vi "uMsg_Delayed Create.vi"(6 "# of times (1)":i32=1, 8 "error in (no error)":errorcluster, 9 "delay (ms)":i32, 10 "Msg":refnum<class "uMsg.lvclass">, 11 "Destination":refnum<class "uTransport.lvclass">) -> (0 "error out":errorcluster, 3 "uMsg_Delayed out":refnum<class "uMsg_Delayed.lvclass">)   [LabVIEW 2023, in "uFramework.lvlib" / "uMsg_Delayed.lvclass"]
uses:
  uMsg_Delayed.lvclass
  uTransport/uTransport.lvclass
  uMsg/uMsg.lvclass
  uMsg_Delayed.lvclass/uMsg_Delayed.ctl
  uMsg_Delayed Daemon.vi
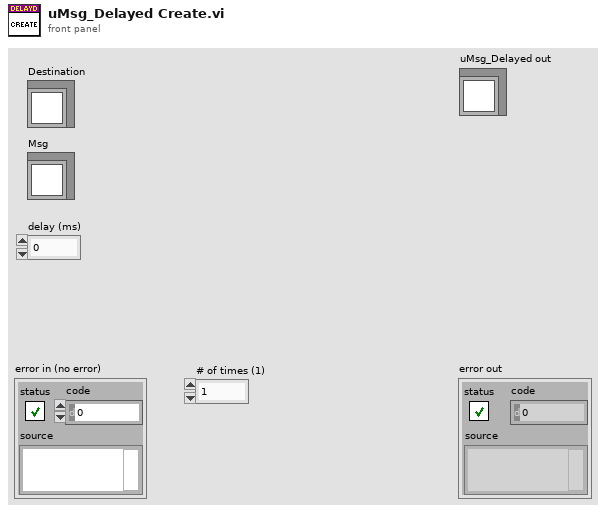
[diagram p1: front panel]
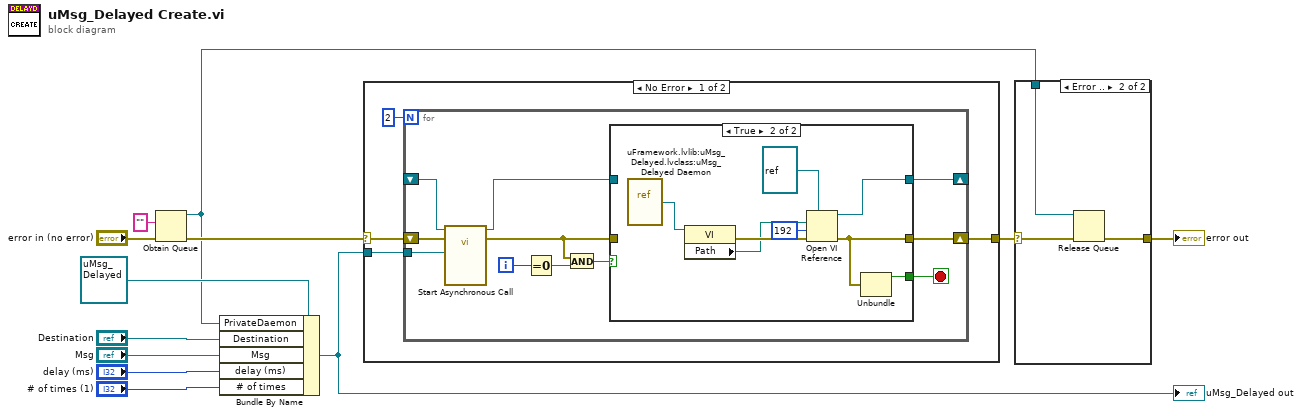
[diagram p0: block diagram]
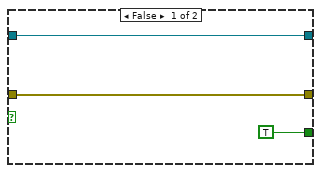
[diagram p3: hidden frame]
diagram:
  n1 = Obtain Queue(element data type="" ("Msg"), error in (no error)="error in (no error)") -> (queue out=w2:refnum<queue>, error out=w12:errorcluster)  [unwired: 3 in, 1 out]
  n2 = Bundle By Name(cluster=refnum<class "uMsg_Delayed.lvclass"> refnum ("uMsg_Delayed in"), "PrivateDaemon"=w2, "Destination"="Destination", "Msg"="Msg", "delay (ms)"="delay (ms)", "# of times"="# of times (1)") -> (w1:refnum<class "uMsg_Delayed.lvclass">)
  "uMsg_Delayed out" <- w1
  n3 = case shown="No Error" w12 {
    selector: w12 -> [w14 w39]
    tunnel: [w16 w39] -> w4
    tunnel: w1 -> [w13 _]
    frame No Error {
      n4 = for {
        N: 2 -> [_]
        shift-right: [w24] -> w16
        shift-left: w14 -> [w27]
        shift-right: [w25] -> _
        shift-left: _ -> [w26]
        tunnel: w13 -> [w17]
        i -> [w23]
        stop <- w18 stop-if-true
        n5 = call-by-ref "Start Asynchronous Call"(reference=w26, error in=w27, "uMsg_Delayed in"=w17) -> (reference out=w22:refnum<vi>, error out=w19:errorcluster)  [unwired: 11 in]
        n6 = Equal To 0?(x=w23) -> (x = 0?=w20:bool)
        n7 = And(x=w19, y=w20) -> (x .and. y?=w21:bool)
        n8 = case shown="True" w21 {
          tunnel: w19 -> [w29 _]
          tunnel: [w30 w34] -> w25
          tunnel: [w29 w33] -> w24
          tunnel: w22 -> [w30 _]
          tunnel: [TRUE w32] -> w18
          frame False {
          }
          frame True {
            n9 = vi-ref "uFramework.lvlib:uMsg_Delayed.lvclass:uMsg_Delayed Daemon.vi"() -> (w35:refnum<vi>)
            n10 = property class="VI"(reference=w35) -> (error out=w38:errorcluster, "Path"=w37:path)  [unwired: 1 in, 1 out]
            n11 = Open VI Reference(type specifier VI Refnum (for type only)=refnum<vi> refnum, vi path=w37, options=192, error in (no error)=w38) -> (vi reference=w34:refnum<vi>, error out=w33:errorcluster)  [unwired: 2 in]
            n12 = Unbundle(w33) -> ("status"=w32:bool)  [unwired: 2 out]
          }
        }
      }
    }
    frame Error {
    }
  }
  n13 = case shown="Error .." w4 {
    selector: w4 -> [w40 w43]
    tunnel: [w40 w42] -> w3
    tunnel: w2 -> [_ w41]
    frame No Error {
    }
    frame Error {
      n14 = Release Queue(queue=w41, error in (no error)=w43) -> (error out=w42:errorcluster)  [unwired: 1 in, 2 out]
    }
  }
  "error out" <- w3
